vi "范例生成.vi"() -> ()   [LabVIEW 2010]
uses:
  <vilib>/DAQmx/read.llb/DAQmx Read.vi
  <vilib>/DAQmx/read.llb/DAQmx Read (Analog 1D Wfm NChan NSamp).vi
  <vilib>/daqmx/miscellaneous.llb/DAQmx Fill In Error Info.vi
panel:
  out "data":waveform(dbl)[](graph) caption="数据"
  in  "stop":bool caption="停止"
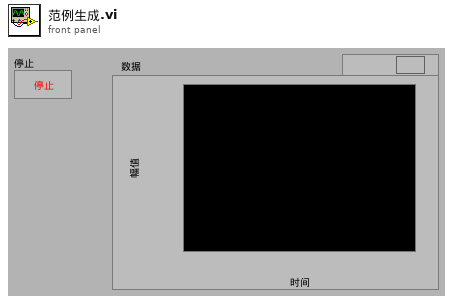
[diagram p1: front panel]
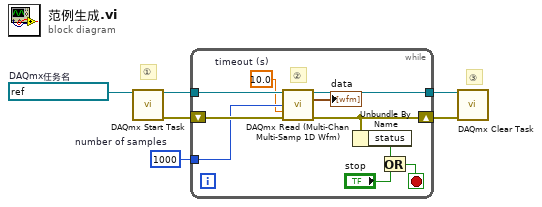
[diagram p0: block diagram]
diagram:
  w4 = 1000  # number of samples
  w1 = refnum<k21> "我的电压任务"  # DAQmx任务名
  # "③"
  # "①"
  n1 = call <vilib>:"DAQmx Start Task.vi"("task/channels in"=w1) -> ("task out"=w6:refnum<k21>, "error out"=w5:errorcluster)  [unwired: 13 in]
  n2 = while "While循环" {
    tunnel: w6 -> [w16]
    tunnel: w4 -> [w12]
    tunnel: [w13] -> w2
    shift-right: [w10] -> w3
    shift-left: w5 -> [w15]
    stop <- w9 stop-if-true
    w7 = 10.0  # timeout (s)
    # "②"
    n3 = call-poly "DAQmx Read (Multi-Chan Multi-Samp 1D Wfm).vi"("task/channels in"=w16, "number of samples per channel"=w12, "timeout"=w7, "error in"=w15) -> ("task out"=w13:refnum<k21>, "data"=→"data":waveform(dbl)[], "error out"=w10:errorcluster)  [unwired: 9 in]
    n4 = Unbundle By Name(w10) -> ("status"=w11:bool)
    n5 = Or(x=w11, y="stop") -> (x .or. y?=w9:bool)
  }
  n6 = call <vilib>:"DAQmx Clear Task.vi"("task in"=w2, "error in"=w3) -> ()  [unwired: 13 in, 1 out]
